vi "Main_Test.vi"() -> ()   [LabVIEW 2023]
uses:
  AFG3022B_class/AFG3022B.lvclass
panel:
  in  "VISA resource name":refnum<visa-resource-name>
  in  "Frequency (1000 Hz)":dbl=1000.0
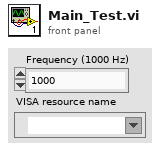
[diagram p1: front panel]
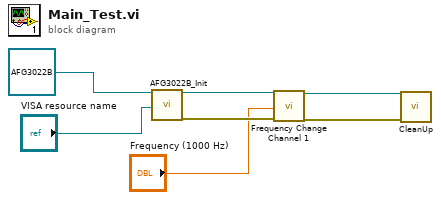
[diagram p0: block diagram]
diagram:
  n1 = call "AFG3022B_Init.vi"("object in"=refnum<class "AFG3022B.lvclass"> refnum, "VISA resource name"="VISA resource name") -> ("object out"=w7:refnum<class "AFG3022B.lvclass">, "error out"=w5:errorcluster)  [unwired: 16 in]
  n2 = call-dynamic "Frequency Change Channel 1.vi"("object in"=w7, "Frequency (1000 Hz)"="Frequency (1000 Hz)", "error in (no error)"=w5) -> ("object out"=w6:refnum<class "AFG3022B.lvclass">, "error out"=w4:errorcluster)  [unwired: 15 in]
  n3 = call-dynamic "CleanUp.vi"("object in"=w6, "error in (no error)"=w4) -> ()  [unwired: 16 in, 2 out]
